vi "FPGA_GlobalReadVersion.vi"(8 "error in (no error)":errorcluster, 11 "GlobalDeviceRef In":T1) -> (0 "error out":errorcluster, 2 "Version":u16=2009, 3 "GlobalDeviceRef Out":T1)   [LabVIEW 2017]
uses:
  <vilib>/Rock Robotics/SystemInterfaces/Global/FPGA_GlobalDevRef.ctl
  <vilib>/Utility/error.llb/Error Cluster From Error Code.vi
  <vilib>/rvi/errors/niLvFpgaAdjustHostInterfaceError.vi
  <vilib>/rvi/interface/nirviReadWriteControl/nirviReadWriteControl.xnode
  <vilib>/Rock Robotics/SystemInterfaces/System/FPGA_SystemFRC FPGA Ref.ctl
  NiFpgaLv.dll
  <vilib>/rvi/interface/Simulation/niFpgaSimulationCallBeginRW.vi
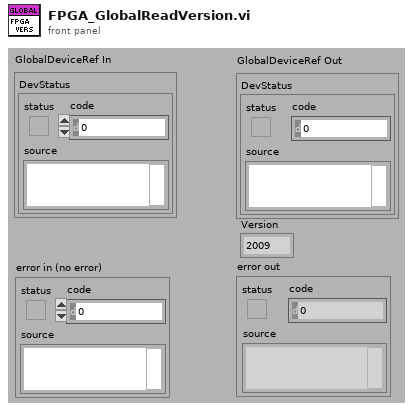
[diagram p1: front panel]
types:
  T1 = typedef "FPGA_GlobalDevRef.ctl" = cluster{"DevStatus":errorcluster}
  T2 = typedef "FPGA_SystemFRC FPGA Ref.ctl" = refnum<k20>
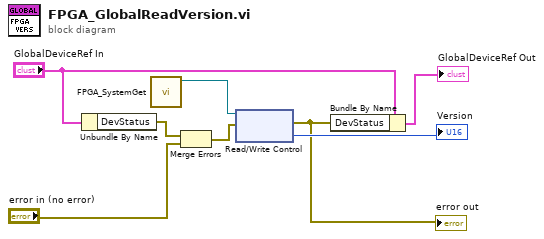
[diagram p0: block diagram]
diagram:
  n1 = Unbundle By Name("GlobalDeviceRef In") -> ("DevStatus"=w4:errorcluster)
  n2 = call <vilib>:"FPGA_SystemGet.vi"() -> ("FRC FPGA Ref"=w1:T2)  [unwired: 11 in]
  n3 = Merge Errors(w4, "error in (no error)") -> (w2:errorcluster)
  n4 = xnode "Read/Write Control"("FPGA VI Reference In"=w1, "error in"=w2) -> ("error out"=w5:errorcluster, "Version"=→"Version":u16)  [unwired: 1 out]
  "error out" <- w5
  n5 = Bundle By Name(cluster="GlobalDeviceRef In", "DevStatus"=w5) -> (→"GlobalDeviceRef Out":T1)
